vi "DisposeApi.vi"(8 "Error in":errorcluster) -> (0 "Error out":errorcluster)   [LabVIEW 2016]
doc: "Use this VI to end the usage of the CommonAPI."
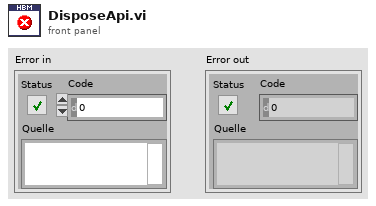
[diagram p1: front panel]
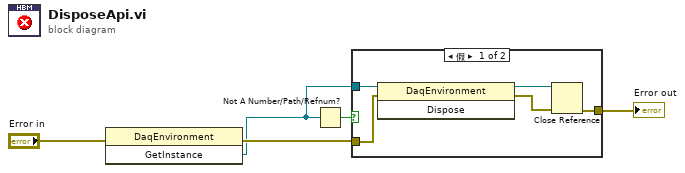
[diagram p0: block diagram]
diagram:
  n1 = invoke on="Methodenknoten" class="DaqEnvironment" method="GetInstance"(error in="Error in") -> (error out=w2:errorcluster, "GetInstance"=w1:refnum<k24>)  [unwired: 2 in, 1 out]
  n2 = Not A Number/Path/Refnum?(number/path/refnum=w1) -> (NaN/Path/Refnum?=w5:bool)
  n3 = case shown="假" w5 {
    tunnel: w1 -> [w10 _]
    tunnel: w2 -> [w7 w11]
    tunnel: [w6 w11] -> w4
    frame False {
      n4 = invoke on="Methodenknoten" class="DaqEnvironment" method="Dispose"(reference=w10, error in=w7) -> (reference out=w9:refnum<k24>, error out=w8:errorcluster)  [unwired: 1 in, 1 out]
      n5 = Close Reference(reference=w9, error in (no error)=w8) -> (error out=w6:errorcluster)
    }
    frame True {
    }
  }
  "Error out" <- w4
